vi "SP Convert Limits Cluster.vi"(4 "Fields Names":string[](array[string]), 5 "Conversion":enum16{"Cluster - HTML", "HTML - Cluster"}(ring), 7 "Limits Key Array In":T7, 8 "Limits Cluster In":T1[](array[typedef]) {"Parameter"."Stimulus Port" min=1 step=1; "Parameter"."Response Port" min=1 step=1}) -> (1 "Limits Cluster Out":T1[](array[typedef]) {"Parameter"."Stimulus Port" min=1 step=1; "Parameter"."Response Port" min=1 step=1}, 2 "Limits HTML Out":string)   [LabVIEW 2011]
uses:
  ITK EXT/utils/keyedarr.llb/Keyed Array.ctl
  TypeDefs/SP Limit.ctl
  TypeDefs/SP Parameter.ctl
  TypeDefs/SP Format.ctl
  TypeDefs/SP Limit Type.ctl
  TypeDefs/SP Limit Point.ctl
  Test Referential Limit.ctl
  ITK EXT/utils/strutil.llb/Case Matching.ctl
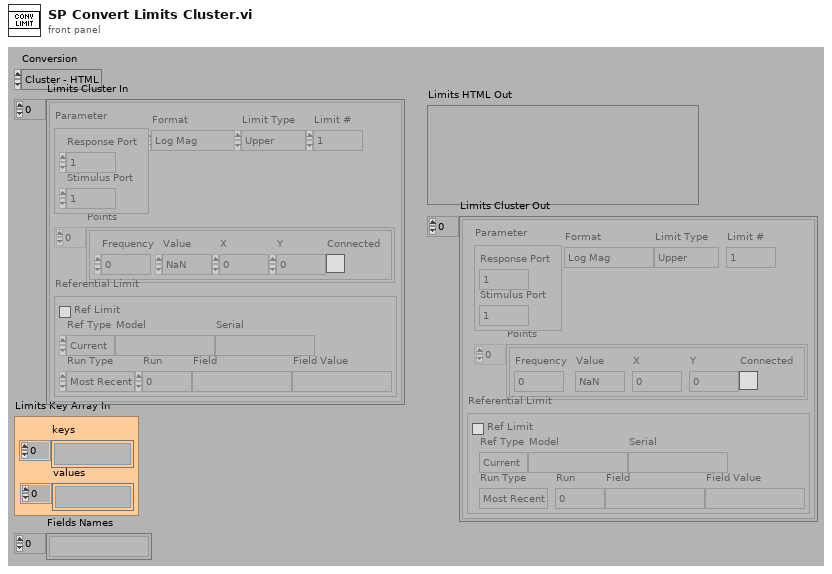
[diagram p1: front panel]
types:
  T1 = typedef "SP Limit.ctl" = cluster{"Parameter":T2, "Format":T3, "Limit Type":T4, "Points":T5[], "Referential Limit":T6, "Limit #":i8}
  T2 = typedef "SP Parameter.ctl" = cluster{"Stimulus Port":i8, "Response Port":i8}
  T3 = typedef "SP Format.ctl" = enum16{"Log Mag", "Lin Mag", "SWR", "Phase", "Expanded Phase", "Delay", "Insertion Loss", "Isolation", "Return Loss"}
  T4 = typedef "SP Limit Type.ctl" = enum16{"Upper", "Lower", "Delta", "Filter", "Referential"}
  T5 = typedef "SP Limit Point.ctl" = cluster{"Frequency":dbl, "Value":dbl, "X":dbl, "Y":dbl, "Connected":bool}
  T6 = typedef "Test Referential Limit.ctl" = cluster{"Ref Limit":bool, "Ref Type":enum16{"Current", "Specify"}, "Model":string, "Serial":string, "Run Type":enum16{"Most Recent", "Run #", "Match Field"}, "Run":i32, "Field":string, "Field Value":string}
  T7 = typedef "Keyed Array.ctl" = cluster{"keys":string[], "values":string[]}
  T8 = typedef "Case Matching.ctl" = enum16{"a != A", "a == A", "system"}
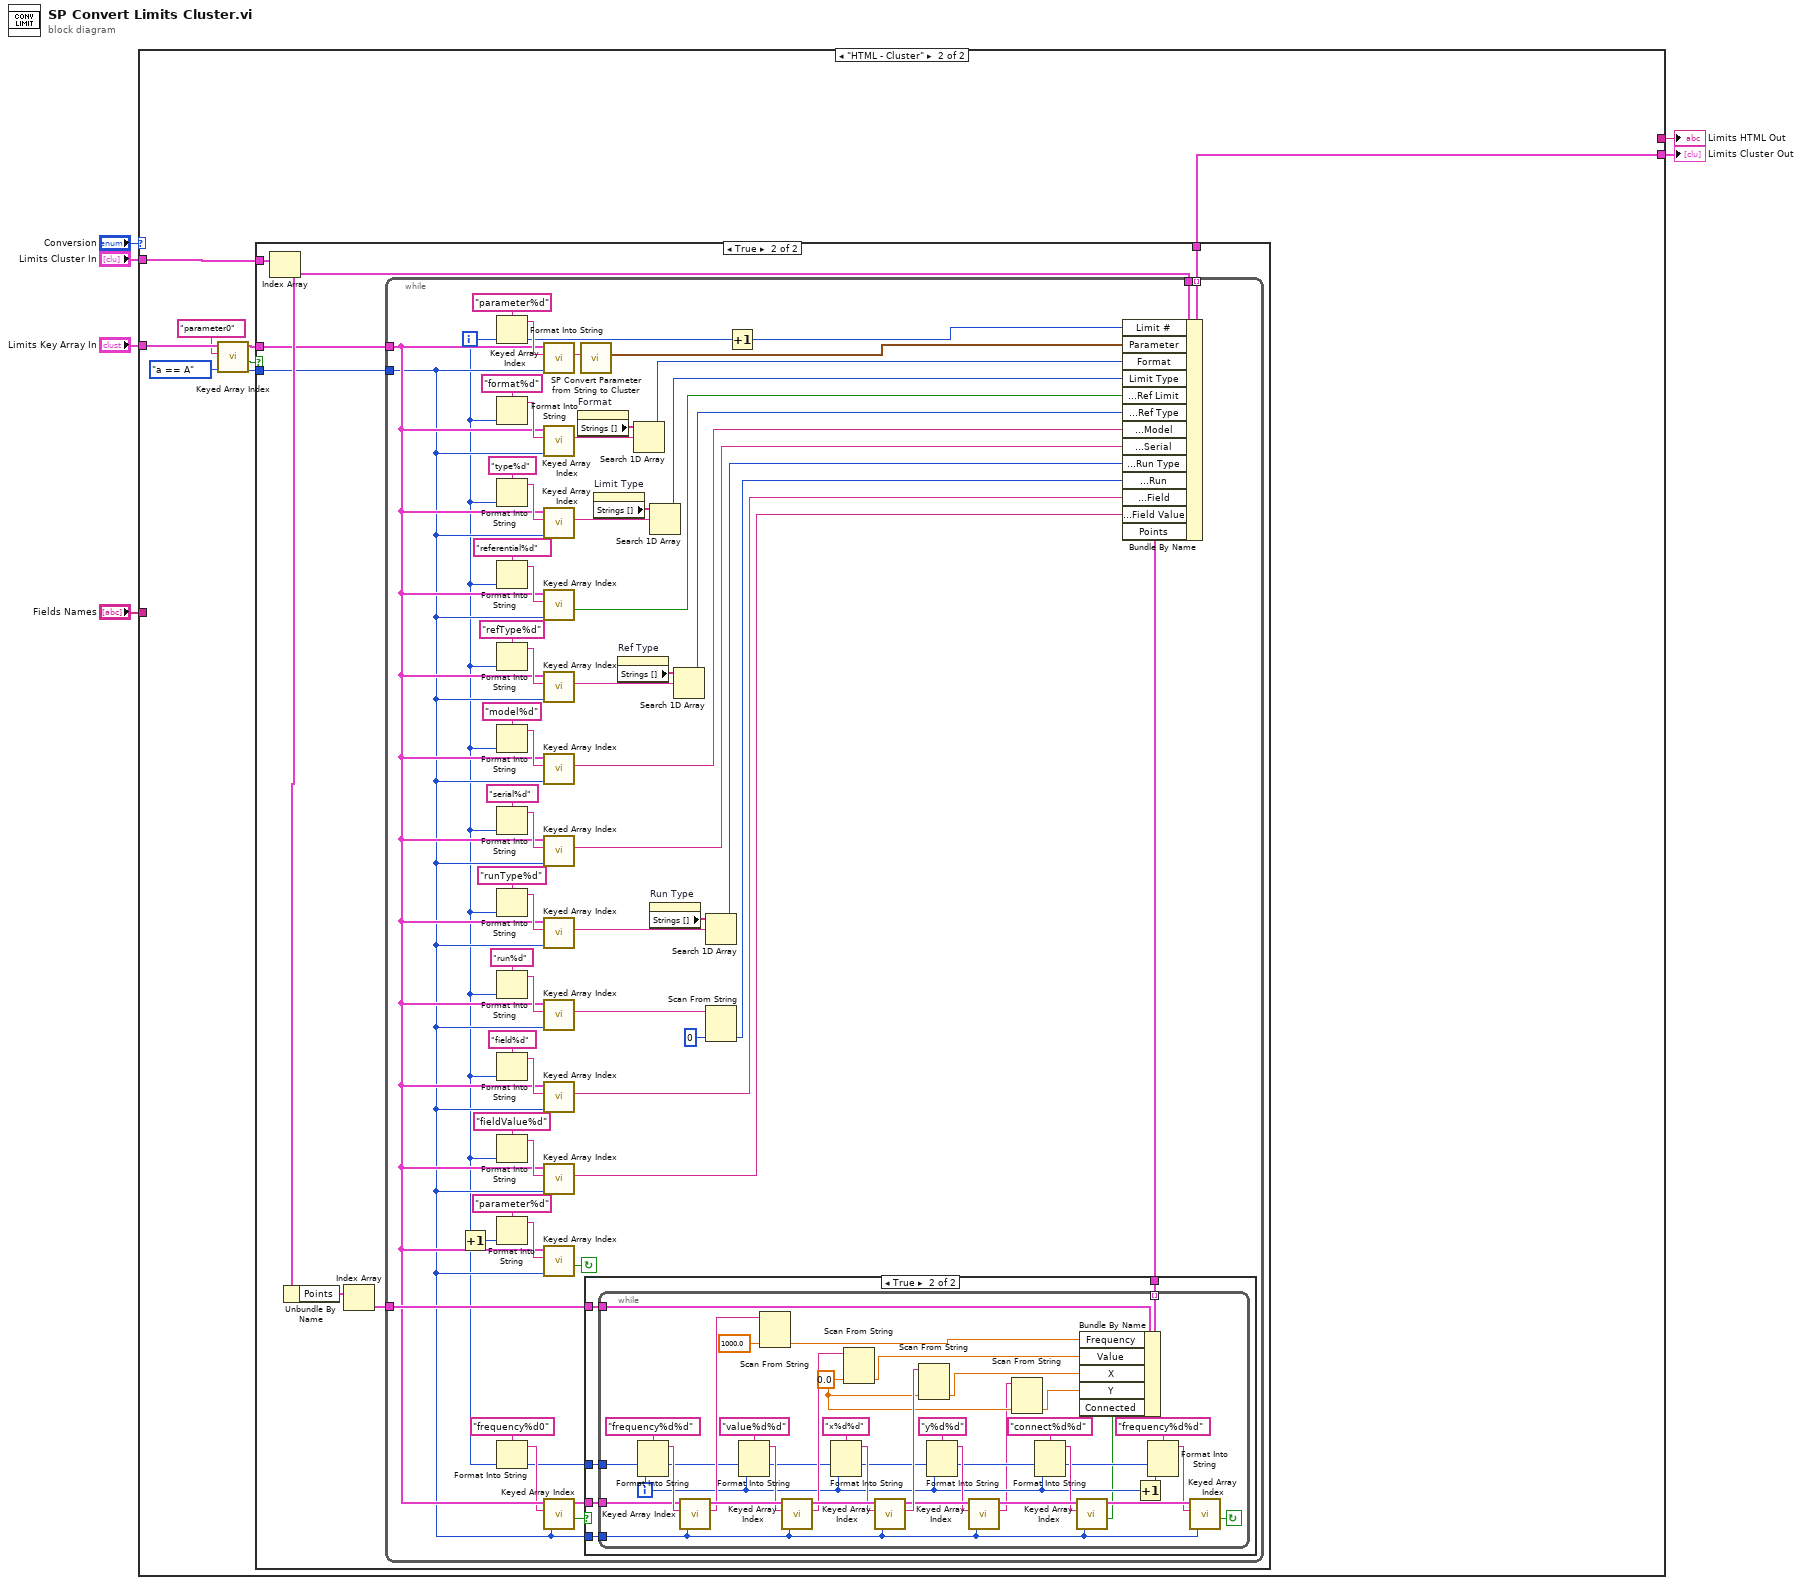
[diagram p0: block diagram]
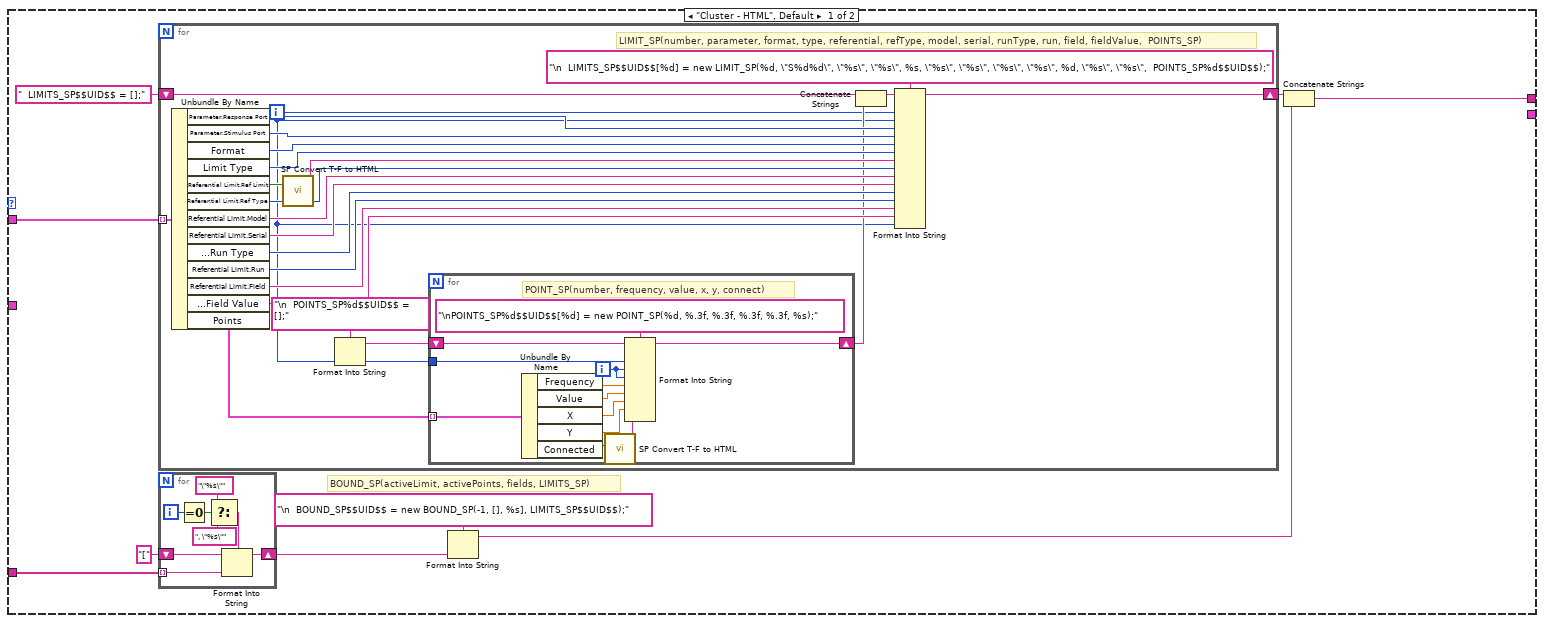
[diagram p2: hidden frame]
diagram:
  n1 = case shown="\"HTML - Cluster\"" "Conversion" {
    tunnel: "Limits Cluster In" -> [w15 w65]
    tunnel: "Limits Key Array In" -> [_ w63]
    tunnel: [w13 _] -> w3
    tunnel: [_ w64] -> w2
    tunnel: "Fields Names" -> [w10 _]
    frame "Cluster - HTML", Default {
      # "BOUND_SP(activeLimit, activePoints, fields, LIMITS_SP)"
      n2 = for {
        tunnel: w15 -> [w46] mode=indexing
        shift-right: [w45] -> w12
        shift-left: "  LIMITS_SP$$UID$$ = [];" ("format string") -> [w27]
        i -> [w24]
        # "LIMIT_SP(number, parameter, format, type, referential, refType, model, serial, runType, run, field, fieldValue,  POINTS_SP)"
        n3 = Unbundle By Name(w46) -> ("Parameter.Response Port"=w41:i8, "Parameter.Stimulus Port"=w40:i8, "Format"=w39:T3, "Limit Type"=w38:T4, "Referential Limit.Ref Limit"=w43:bool, "Referential Limit.Ref Type"=w36:enum16{"Current", "Specify"}, "Referential Limit.Model"=w35:string, "Referential Limit.Serial"=w34:string, "Referential Limit.Run Type"=w33:enum16{"Most Recent", "Run #", "Match Field"}, "Referential Limit.Run"=w32:i32, "Referential Limit.Field"=w31:string, "Referential Limit.Field Value"=w30:string, "Points"=w42:T5[])
        n4 = call "SP Convert T-F to HTML.vi"("(T/F)"=w43) -> ("HTML (true/false)"=w37:string)  [unwired: 10 out]
        n5 = Format Into String(format string="\n  POINTS_SP%d$$UID$$ = [];", w24) -> (resulting string=w28:string)  [unwired: 2 in, 1 out]
        n6 = for {
          tunnel: w42 -> [w58] mode=indexing
          shift-right: [w53] -> w25
          shift-left: w28 -> [w52]
          tunnel: w24 -> [w47]
          i -> [w51]
          # "POINT_SP(number, frequency, value, x, y, connect)"
          n7 = Unbundle By Name(w58) -> ("Frequency"=w55:dbl, "Value"=w54:dbl, "X"=w56:dbl, "Y"=w50:dbl, "Connected"=w48:bool)
          n8 = call "SP Convert T-F to HTML.vi"("(T/F)"=w48) -> ("HTML (true/false)"=w49:string)  [unwired: 10 out]
          n9 = Format Into String(format string="\nPOINTS_SP%d$$UID$$[%d] = new POINT_SP(%d, %.3f, %.3f, %.3f, %.3f, %s);", initial string=w52, w47, w51, w51, w55, w54, w56, w50, w49) -> (resulting string=w53:string)  [unwired: 1 in, 1 out]
        }
        n10 = Concatenate Strings(w27, w25) -> (w26:string)
        n11 = Format Into String(format string="\n  LIMITS_SP$$UID$$[%d] = new LIMIT_SP(%d, \"S%d%d\", \"%s\", \"%s\", %s, \"%s\", \"%s\", \"%s\", \"%s\", %d, \"%s\", \"%s\",  POINTS_SP%d$$UID$$);", initial string=w26, w24, w24, w41, w40, w39, w38, w37, w36, w35, w34, w33, w32, w31, w30, w24) -> (resulting string=w45:string)  [unwired: 1 in, 1 out]
      }
      n12 = for {
        shift-right: [w16] -> w8
        shift-left: "[" ("format string") -> [w23]
        tunnel: w10 -> [w17] mode=indexing
        i -> [w22]
        n13 = Equal To 0?(x=w22) -> (x = 0?=w21:bool)
        n14 = Select(t="\"%s\"" ("format string"), s=w21, f=", \"%s\"" ("format string")) -> (s? t:f=w18:string)
        n15 = Format Into String(format string=w18, initial string=w23, w17) -> (resulting string=w16:string)  [unwired: 1 in, 1 out]
      }
      n16 = Format Into String(format string="\n  BOUND_SP$$UID$$ = new BOUND_SP(-1, [], %s], LIMITS_SP$$UID$$);", w8) -> (resulting string=w7:string)  [unwired: 2 in, 1 out]
      n17 = Concatenate Strings(w12, w7) -> (w13:string)
    }
    frame "HTML - Cluster" {
      w60 = Case_Matching."a == A" ("case matching (sensitive)")
      n18 = call "Keyed Array Index.vi"("case matching (sensitive)"=w60, "key"="parameter0", "array in"=w63) -> ("valid key"=w59:bool, "duplicate array"=w62:T7)  [unwired: 1 in, 2 out]
      n19 = case shown="True" w59 {
        tunnel: w65 -> [_ w72]
        tunnel: [_ w71] -> w64
        tunnel: w62 -> [_ w67]
        tunnel: w60 -> [_ w66]
        frame False {
        }
        frame True {
          n20 = Index Array(array=w72) -> (element=w69:T1)  [unwired: 1 in]
          n21 = Unbundle By Name(w69) -> ("Points"=w70:T5[])
          n22 = Index Array(array=w70) -> (element=w68:T5)  [unwired: 1 in]
          n23 = while {
            tunnel: w69 -> [w132]
            tunnel: [w131] -> w71 mode=indexing
            tunnel: w67 -> [w79]
            tunnel: w68 -> [w129]
            tunnel: w66 -> [w78]
            i -> [w74]
            stop <- w81 continue-if-true
            n24 = Increment(x=w74) -> (x+1=w82:i32)
            n25 = Format Into String(format string="parameter%d", w74) -> (resulting string=w128:string)  [unwired: 2 in, 1 out]
            n26 = Format Into String(format string="format%d", w74) -> (resulting string=w124:string)  [unwired: 2 in, 1 out]
            n27 = Format Into String(format string="type%d", w74) -> (resulting string=w121:string)  [unwired: 2 in, 1 out]
            n28 = Format Into String(format string="referential%d", w74) -> (resulting string=w120:string)  [unwired: 2 in, 1 out]
            n29 = Format Into String(format string="refType%d", w74) -> (resulting string=w117:string)  [unwired: 2 in, 1 out]
            n30 = Format Into String(format string="model%d", w74) -> (resulting string=w116:string)  [unwired: 2 in, 1 out]
            n31 = Format Into String(format string="serial%d", w74) -> (resulting string=w113:string)  [unwired: 2 in, 1 out]
            n32 = Format Into String(format string="runType%d", w74) -> (resulting string=w112:string)  [unwired: 2 in, 1 out]
            n33 = Format Into String(format string="run%d", w74) -> (resulting string=w109:string)  [unwired: 2 in, 1 out]
            n34 = Format Into String(format string="field%d", w74) -> (resulting string=w108:string)  [unwired: 2 in, 1 out]
            n35 = Format Into String(format string="fieldValue%d", w74) -> (resulting string=w105:string)  [unwired: 2 in, 1 out]
            n36 = Format Into String(format string="parameter%d", w82) -> (resulting string=w84:string)  [unwired: 2 in, 1 out]
            n37 = Format Into String(format string="frequency%d0", w74) -> (resulting string=w76:string)  [unwired: 2 in, 1 out]
            n38 = call "Keyed Array Index.vi"("case matching (sensitive)"=w78, "key"=w128, "array in"=w79) -> ("value"=w126:string)  [unwired: 1 in, 3 out]
            n39 = call "Keyed Array Index.vi"("case matching (sensitive)"=w78, "key"=w124, "array in"=w79) -> ("value"=w103:string)  [unwired: 1 in, 3 out]
            n40 = call "Keyed Array Index.vi"("case matching (sensitive)"=w78, "key"=w121, "array in"=w79) -> ("value"=w100:string)  [unwired: 1 in, 3 out]
            n41 = call "Keyed Array Index.vi"("case matching (sensitive)"=w78, "key"=w120, "array in"=w79) -> ("valid key"=w98:bool)  [unwired: 1 in, 3 out]
            n42 = call "Keyed Array Index.vi"("case matching (sensitive)"=w78, "key"=w117, "array in"=w79) -> ("value"=w96:string)  [unwired: 1 in, 3 out]
            n43 = call "Keyed Array Index.vi"("case matching (sensitive)"=w78, "key"=w116, "array in"=w79) -> ("value"=w94:string)  [unwired: 1 in, 3 out]
            n44 = call "Keyed Array Index.vi"("case matching (sensitive)"=w78, "key"=w113, "array in"=w79) -> ("value"=w93:string)  [unwired: 1 in, 3 out]
            n45 = call "Keyed Array Index.vi"("case matching (sensitive)"=w78, "key"=w112, "array in"=w79) -> ("value"=w91:string)  [unwired: 1 in, 3 out]
            n46 = call "Keyed Array Index.vi"("case matching (sensitive)"=w78, "key"=w109, "array in"=w79) -> ("value"=w89:string)  [unwired: 1 in, 3 out]
            n47 = call "Keyed Array Index.vi"("case matching (sensitive)"=w78, "key"=w108, "array in"=w79) -> ("value"=w86:string)  [unwired: 1 in, 3 out]
            n48 = call "Keyed Array Index.vi"("case matching (sensitive)"=w78, "key"=w105, "array in"=w79) -> ("value"=w85:string)  [unwired: 1 in, 3 out]
            n49 = call "Keyed Array Index.vi"("case matching (sensitive)"=w78, "key"=w84, "array in"=w79) -> ("valid key"=w81:bool)  [unwired: 1 in, 3 out]
            n50 = call "Keyed Array Index.vi"("case matching (sensitive)"=w78, "key"=w76, "array in"=w79) -> ("valid key"=w75:bool, "duplicate array"=w77:T7)  [unwired: 1 in, 2 out]
            n51 = property on="Format" class="Enum (strict)"() -> ("Strings []"=w104:string[])  [unwired: 2 in, 2 out]
            n52 = call "SP Convert Parameter from String to Cluster.vi"("Parameter String"=w126) -> ("Parameter"=w125:T2)  [unwired: 10 out]
            n53 = case shown="True" w75 {
              tunnel: w129 -> [_ w137]
              tunnel: [_ w136] -> w127
              tunnel: w78 -> [_ w135]
              tunnel: w77 -> [_ w134]
              tunnel: w74 -> [_ w133]
              frame False {
              }
              frame True {
                n54 = while {
                  tunnel: w137 -> [w169]
                  tunnel: [w168] -> w136 mode=indexing
                  tunnel: w135 -> [w147]
                  tunnel: w134 -> [w153]
                  tunnel: w133 -> [w145]
                  i -> [w146]
                  stop <- w138 continue-if-true
                  w141 = 0.0 ("default value 1")
                  n55 = Format Into String(format string="frequency%d%d", w145, w146) -> (resulting string=w166:string)  [unwired: 2 in, 1 out]
                  n56 = call "Keyed Array Index.vi"("case matching (sensitive)"=w147, "key"=w166, "array in"=w153) -> ("value"=w165:string, "duplicate array"=w170:T7)  [unwired: 1 in, 2 out]
                  n57 = Format Into String(format string="value%d%d", w145, w146) -> (resulting string=w161:string)  [unwired: 2 in, 1 out]
                  n58 = Scan From String(input string=w165, default 1=1000.0 ("default value 1")) -> (output 1=w164:dbl)  [unwired: 3 in, 3 out]
                  n59 = call "Keyed Array Index.vi"("case matching (sensitive)"=w147, "key"=w161, "array in"=w170) -> ("value"=w159:string, "duplicate array"=w171:T7)  [unwired: 1 in, 2 out]
                  n60 = Format Into String(format string="x%d%d", w145, w146) -> (resulting string=w160:string)  [unwired: 2 in, 1 out]
                  n61 = Scan From String(input string=w159, default 1=w141) -> (output 1=w158:dbl)  [unwired: 3 in, 3 out]
                  n62 = call "Keyed Array Index.vi"("case matching (sensitive)"=w147, "key"=w160, "array in"=w171) -> ("value"=w157:string, "duplicate array"=w155:T7)  [unwired: 1 in, 2 out]
                  n63 = Scan From String(input string=w157, default 1=w141) -> (output 1=w143:dbl)  [unwired: 3 in, 3 out]
                  n64 = Format Into String(format string="y%d%d", w145, w146) -> (resulting string=w154:string)  [unwired: 2 in, 1 out]
                  n65 = call "Keyed Array Index.vi"("case matching (sensitive)"=w147, "key"=w154, "array in"=w155) -> ("value"=w140:string, "duplicate array"=w173:T7)  [unwired: 1 in, 2 out]
                  n66 = Scan From String(input string=w140, default 1=w141) -> (output 1=w142:dbl)  [unwired: 3 in, 3 out]
                  n67 = Format Into String(format string="connect%d%d", w145, w146) -> (resulting string=w152:string)  [unwired: 2 in, 1 out]
                  n68 = call "Keyed Array Index.vi"("case matching (sensitive)"=w147, "key"=w152, "array in"=w173) -> ("valid key"=w139:bool, "duplicate array"=w172:T7)  [unwired: 1 in, 2 out]
                  n69 = Bundle By Name(cluster=w169, "Frequency"=w164, "Value"=w158, "X"=w143, "Y"=w142, "Connected"=w139) -> (w168:T5)
                  n70 = Increment(x=w146) -> (x+1=w149:i32)
                  n71 = Format Into String(format string="frequency%d%d", w145, w149) -> (resulting string=w148:string)  [unwired: 2 in, 1 out]
                  n72 = call "Keyed Array Index.vi"("case matching (sensitive)"=w147, "key"=w148, "array in"=w172) -> ("valid key"=w138:bool)  [unwired: 1 in, 3 out]
                }
              }
            }
            n73 = property on="Limit Type" class="Enum (strict)"() -> ("Strings []"=w101:string[])  [unwired: 2 in, 2 out]
            n74 = property on="Ref Type" class="Enum (strict)"() -> ("Strings []"=w97:string[])  [unwired: 2 in, 2 out]
            n75 = Search 1D Array(1D array=w104, element=w103) -> (index of element=w102:i32)  [unwired: 1 out]
            n76 = Search 1D Array(1D array=w101, element=w100) -> (index of element=w99:i32)  [unwired: 1 out]
            n77 = property on="Run Type" class="Enum (strict)"() -> ("Strings []"=w92:string[])  [unwired: 2 in, 2 out]
            n78 = Search 1D Array(1D array=w97, element=w96) -> (index of element=w95:i32)  [unwired: 1 out]
            n79 = Search 1D Array(1D array=w92, element=w91) -> (index of element=w90:i32)  [unwired: 1 out]
            n80 = Scan From String(input string=w89, default 1=0 ("default value 1")) -> (output 1=w88:i32)  [unwired: 3 in, 3 out]
            n81 = Increment(x=w74) -> (x+1=w73:i32)
            n82 = Bundle By Name(cluster=w132, "Limit #"=w73, "Parameter"=w125, "Format"=w102, "Limit Type"=w99, "Referential Limit.Ref Limit"=w98, "Referential Limit.Ref Type"=w95, "Referential Limit.Model"=w94, "Referential Limit.Serial"=w93, "Referential Limit.Run Type"=w90, "Referential Limit.Run"=w88, "Referential Limit.Field"=w86, "Referential Limit.Field Value"=w85, "Points"=w127) -> (w131:T1)
          }
        }
      }
    }
  }
  "Limits HTML Out" <- w3
  "Limits Cluster Out" <- w2
